vi "VisualizePmuResults.vi"() -> ()   [LabVIEW 2018, in "Visualization.lvlib" / "VisualizeAnalysis.lvclass"]
uses:
  VisualizeAnalysis.lvclass
  VisualizeBase/VisualizeBase_class/Requests/VisUserEventType.ctl
  <vilib>/event_ctls.llb/usereventprio.ctl
  <vilib>/Utility/file.llb/Read From Spreadsheet File (DBL).vi
  <vilib>/Utility/error.llb/Error Cluster From Error Code.vi
  <vilib>/ErrorRing/Error Ring.xnode
  VisualizeBase/VisualizeBase_class/VisualizeBase.lvclass
  <userlib>/NIST/NISTErrorLib/NISTErrorLib.lvlib
  Analysis/AnalysisModule/AnalysisModule.lvlib
  Visualization.lvlib
panel:
  in  "btnReset":bool
  in  "btnClear":bool
  in  "Pause":bool
  out "Data from file":dbl[][](array[numeric])
  in  "btnOpen":bool
  out "RFE":dbl(graph)=-0.0019269131938461162
  out "FE":dbl(graph)=1.1347977483922023e-05
  out "Data real time":dbl[](array[numeric])
  out "TVE":cluster{timestamp[], dbl[]}[](graph)
  in  "QueName":string="AnalVisQue"
  out "ErrorArray":errorcluster[](array[cluster])
  in  "btnStop":bool
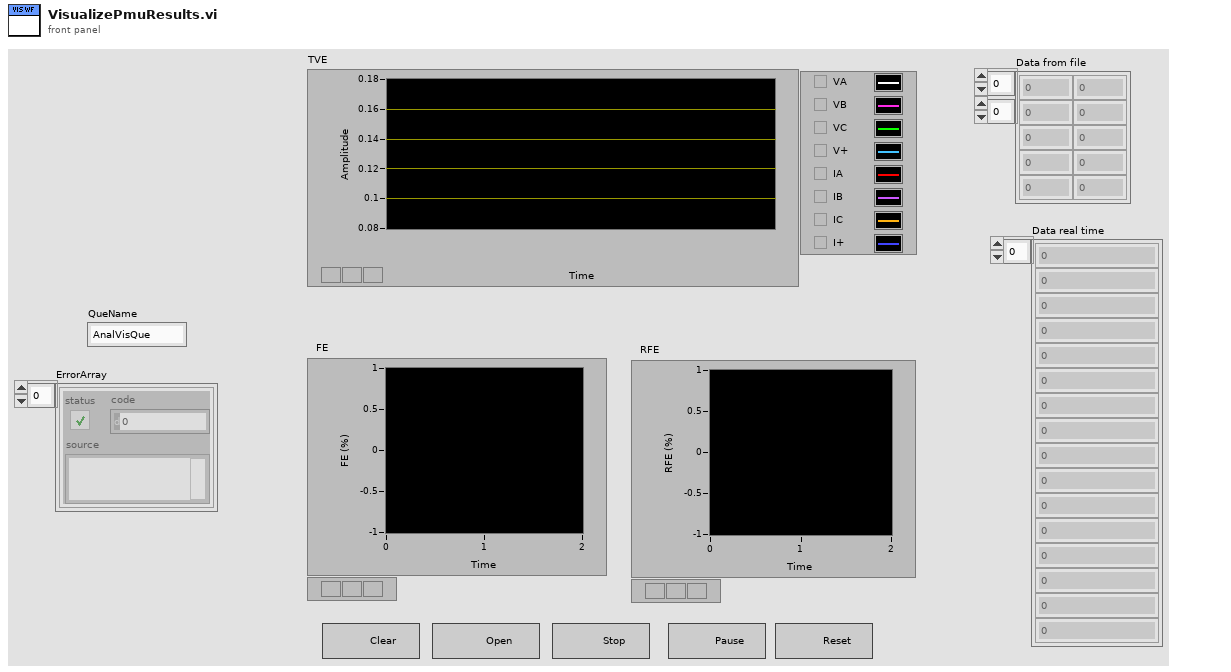
[diagram p1: front panel]
types:
  T1 = typedef "Visualization.lvlib/VisualizeBase.lvclass/VisRequestEvents.ctl" = cluster{"StopRequest":refnum<user-event>, "ResetRequest":refnum<user-event>, "FP Pop In or Out":refnum<user-event>}
  T2 = typedef "AnalysisModule.lvlib/clBroadcastEvents.ctl" = cluster{"DidInit":refnum<user-event>, "StatusUpdate":refnum<user-event>, "ErrorReport":refnum<user-event>, "DidStop":refnum<user-event>, "PathToINI":refnum<user-event>, "Config":refnum<user-event>, "ResultReport":refnum<user-event>, "FunctionClass":refnum<user-event>, "State":refnum<user-event>, "FunctionParams":refnum<user-event>, "Duration":refnum<user-event>}
  T3 = typedef "Visualization.lvlib/VisualizeBase.lvclass/VisUserEventType.ctl" = cluster{"BusIndex":i8, "Data":variant}
  T4 = typedef "usereventprio.ctl" = enum32{"high priority", "normal priority"}
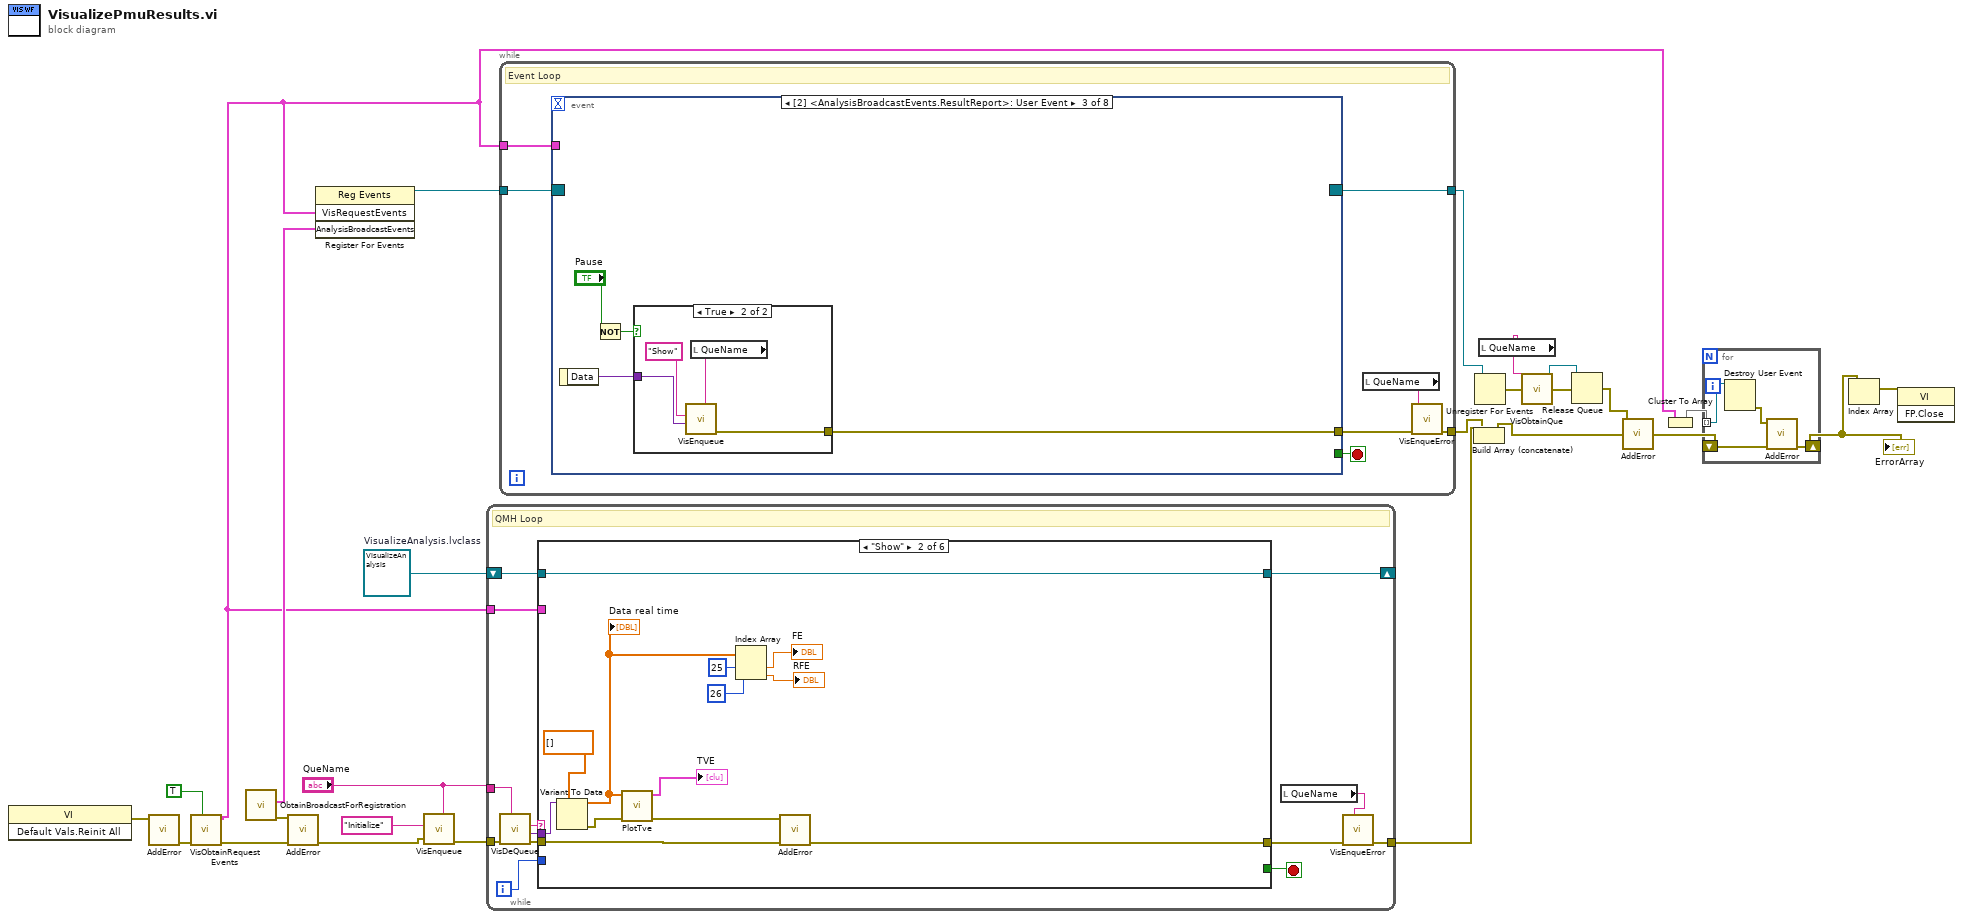
[diagram p0: block diagram]
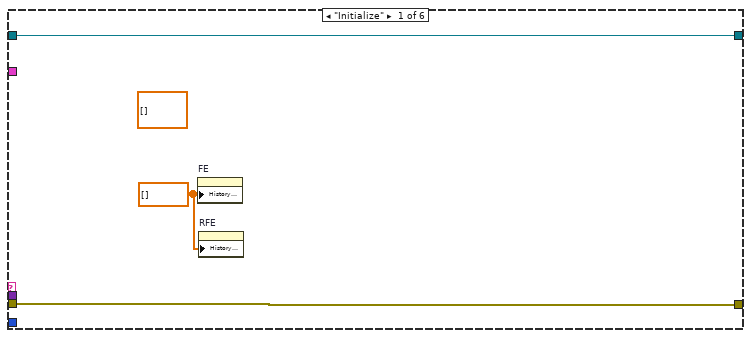
[diagram p2: hidden frame]
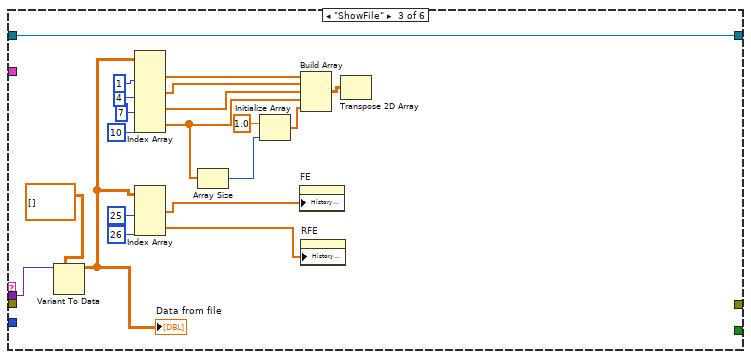
[diagram p3: hidden frame]
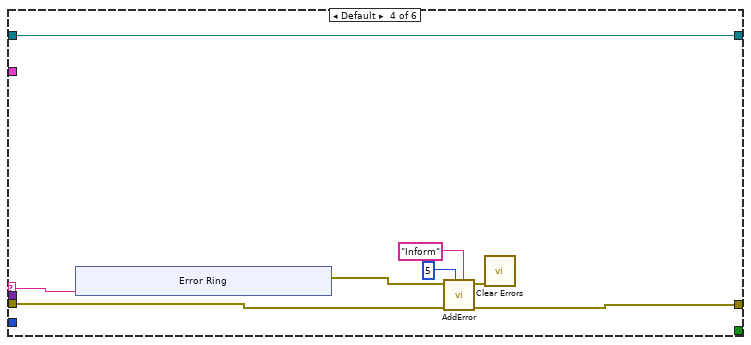
[diagram p4: hidden frame]
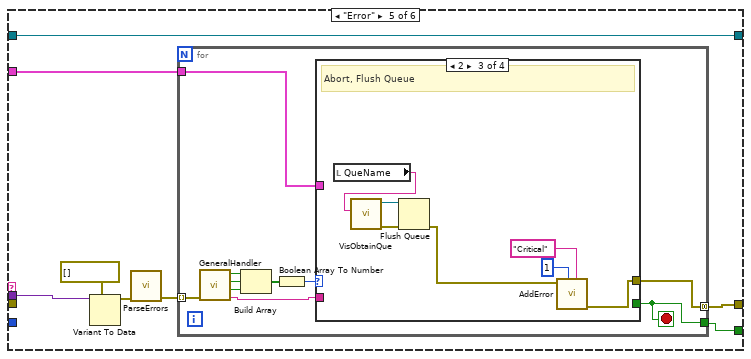
[diagram p5: hidden frame]
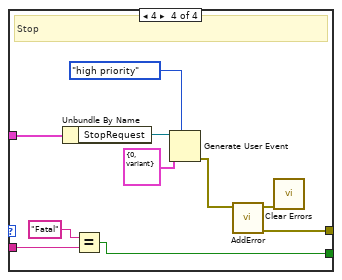
[diagram p8: hidden frame]
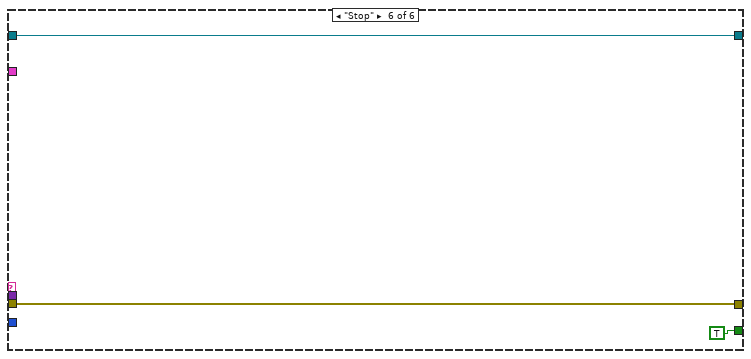
[diagram p9: hidden frame]
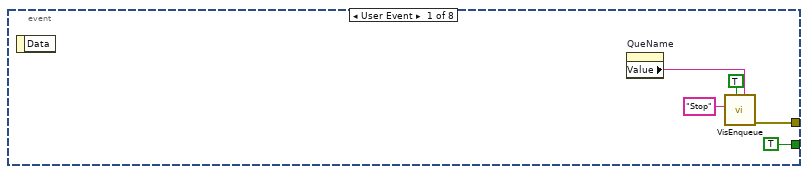
[diagram p10: hidden frame]
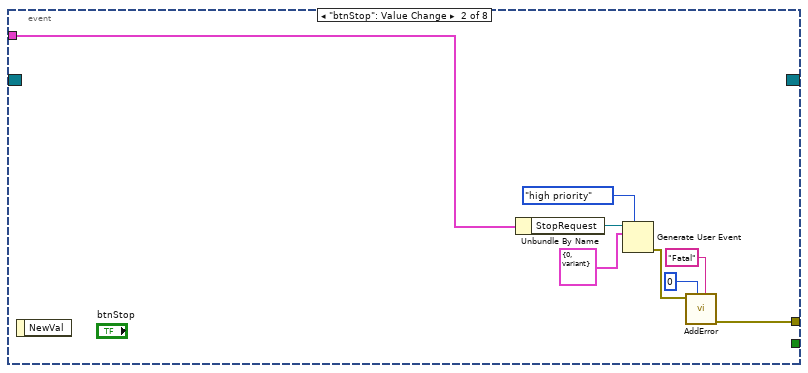
[diagram p11: hidden frame]
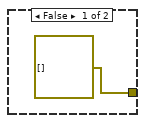
[diagram p12: hidden frame]
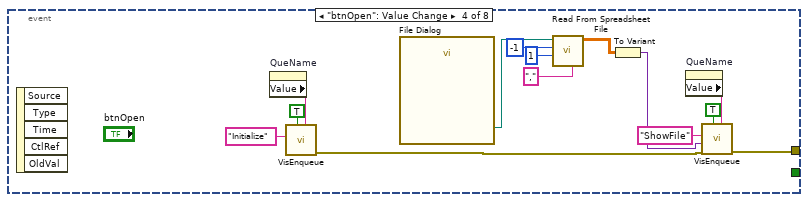
[diagram p13: hidden frame]
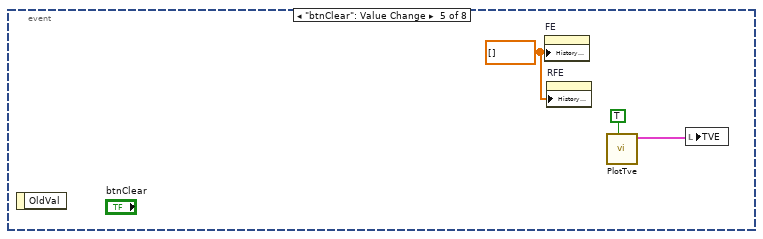
[diagram p14: hidden frame]
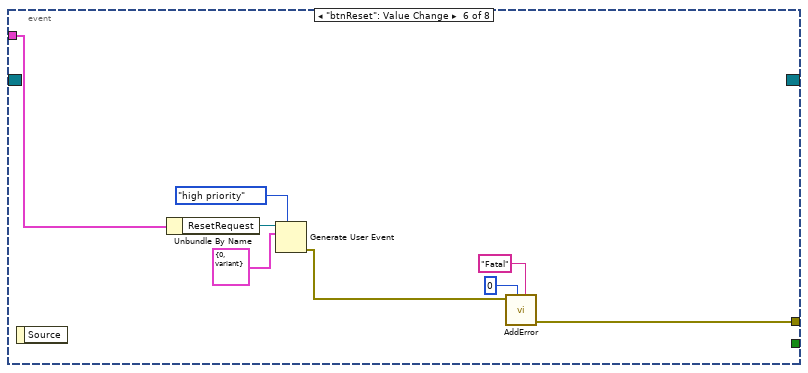
[diagram p15: hidden frame]
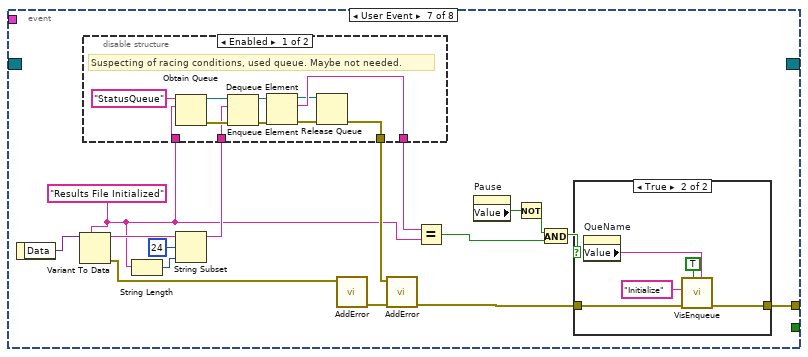
[diagram p16: hidden frame]
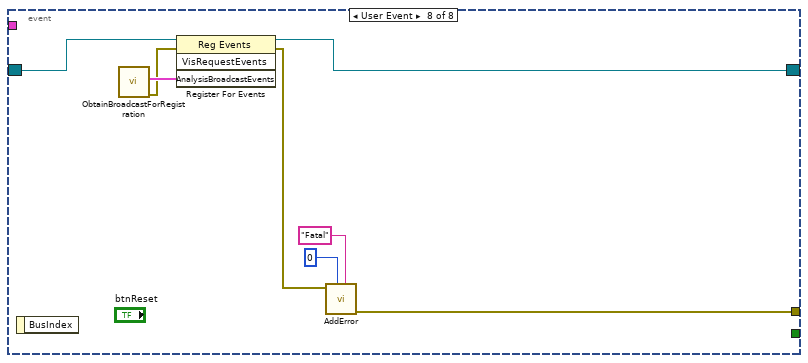
[diagram p19: hidden frame]
diagram:
  w15 = refnum<class "VisualizeAnalysis.lvclass"> refnum  # VisualizeAnalysis.lvclass
  n1 = invoke class="VI" method="Default Vals.Reinit All"() -> (error out=w22:errorcluster)  [unwired: 3 in, 2 out]
  n2 = call <userlib>:"AddError.vi"("error in (no error)"=w22) -> ("ErrorArray Out"=w21:errorcluster[])  [unwired: 9 in, 1 out]
  n3 = call "VisObtainRequestEvents.vi"("Set (T)/Get (F)"=TRUE, "Error"=w21) -> ("Error"=w19:errorcluster[], "VisRequestEvents"=w2:T1)  [unwired: 8 in]
  n4 = call "ObtainBroadcastForRegistration.vi"() -> ("error out"=w17:errorcluster, "AnalysisBroadcastEvents"=w20:T2)  [unwired: 10 in]
  n5 = call <userlib>:"AddError.vi"("ErrorArray In"=w19, "error in (no error)"=w17) -> ("ErrorArray Out"=w18:errorcluster[])  [unwired: 8 in, 1 out]
  n6 = register-events(w2, w20) -> (reference out=w14:refnum<event-registration>)  [unwired: 2 in, 1 out]
  n7 = call "VisEnqueue.vi"("QueName"="QueName", "Error"=w18, "Message"="Initialize") -> ("Error"=w25:errorcluster[])  [unwired: 8 in]
  n8 = while {
    tunnel: w25 -> [w39]
    tunnel: [w33] -> w24
    tunnel: "QueName" -> [w31]
    shift-right: [w30] -> _
    shift-left: w15 -> [w29]
    tunnel: w2 -> [w28]
    i -> [w27]
    stop <- w34 stop-if-true
    # "QMH Loop"
    n9 = call "VisDeQueue.vi"("QueName"=w31, "Error"=w39) -> ("Error"=w36:errorcluster[], "Data"=w37:variant, "Message"=w38:string)  [unwired: 7 in]
    n10 = case shown="\"Show\"" w38 {
      selector: w38 -> [_ _ _ w83 _ _]
      tunnel: w37 -> [_ w54 w75 _ w98 _]
      tunnel: w36 -> [w42 w49 _ w81 _ w127]
      tunnel: [w42 w48 _ w80 w94 w127] -> w35
      tunnel: [_ _ _ _ w93 TRUE] -> w34
      tunnel: w29 -> [w41 w55 w73 w76 w92 w126]
      tunnel: [w41 w55 w73 w76 w92 w126] -> w30
      tunnel: w28 -> [_ _ _ _ w91 _]
      tunnel: w27 -> [_ _ _ _ _ _]
      frame "Initialize" {
        w40 = dbl[] [] ("History Data")
        (unwired) dbl[][] [] ("History Data")
        n11 = property on="FE" class="WFChart (strict)"("History Data"=w40) -> ()  [unwired: 2 in, 2 out]
        n12 = property on="RFE" class="WFChart (strict)"("History Data"=w40) -> ()  [unwired: 2 in, 2 out]
      }
      frame "Show" {
        n13 = Variant To Data(type=dbl[] [], Variant=w54) -> (data=w45:dbl[], error out=w47:errorcluster)  [unwired: 1 in]
        "Data real time" <- w45
        n14 = call "PlotTve.vi"("error in (no error)"=w47, "Data real time"=w45) -> ("error out"=w46:errorcluster, "TVE"=→"TVE":cluster{timestamp[], dbl[]}[])  [unwired: 8 in]
        n15 = Index Array(array=w45, index #1=25 ("index"), index #2=26 ("index")) -> (element #1=→"FE":dbl, element #2=→"RFE":dbl)
        n16 = call <userlib>:"AddError.vi"("ErrorArray In"=w49, "error in (no error)"=w46) -> ("ErrorArray Out"=w48:errorcluster[])  [unwired: 8 in, 1 out]
      }
      frame "ShowFile" {
        n17 = Variant To Data(type=dbl[][] [], Variant=w75) -> (data=w64:dbl[][])  [unwired: 1 in, 1 out]
        "Data from file" <- w64
        n18 = Index Array(array=w64, index (col) #1=1 ("disabled index (col)"), index (col) #2=4 ("index (col)"), index (col) #3=7 ("index (col)"), index (col) #4=10 ("index (col)")) -> (element #1=w68:dbl[], element #2=w67:dbl[], element #3=w66:dbl[], element #4=w59:dbl[])  [unwired: 4 in]
        n19 = Index Array(array=w64, index (col) #1=25 ("disabled index (col)"), index (col) #2=26 ("index (col)")) -> (element #1=w61:dbl[], element #2=w60:dbl[])  [unwired: 2 in]
        n20 = Array Size(array=w59) -> (size(s)=w58:i32)
        n21 = Initialize Array(1.0 ("element"), w58) -> (w56:dbl[])
        n22 = property on="FE" class="WFChart (strict)"("History Data"=w61) -> ()  [unwired: 2 in, 2 out]
        n23 = Build Array(w68, w67, w66, w59, w56) -> (w65:dbl[][])
        n24 = property on="RFE" class="WFChart (strict)"("History Data"=w60) -> ()  [unwired: 2 in, 2 out]
        n25 = Transpose 2D Array(2D array=w65) -> ()  [unwired: 1 out]
      }
      frame Default {
        n26 = xnode "Error Ring"("parameter 0"=w83) -> ("error out"=w82:errorcluster)
        n27 = call <userlib>:"AddError.vi"("Severity"="Inform" ("String"), "Priority"=u8 5, "ErrorArray In"=w81, "error in (no error)"=w82) -> ("ErrorArray Out"=w80:errorcluster[], "error out"=w79:errorcluster)  [unwired: 6 in]
        n28 = call <vilib>:"Clear Errors.vi"("error in (no error)"=w79) -> ()  [unwired: 5 in, 2 out]
      }
      frame "Error" {
        n29 = Variant To Data(type=errorcluster[] [], Variant=w98) -> (data=w96:errorcluster[])  [unwired: 1 in, 1 out]
        n30 = call <userlib>:"ParseErrors.vi"("ErrorArray"=w96) -> ("ErrorArray"=w95:errorcluster[])  [unwired: 8 in, 2 out]
        n31 = for {
          tunnel: w95 -> [w108] mode=indexing
          tunnel: [w102] -> w94 mode=concatenating
          tunnel: [w100] -> w93
          tunnel: w91 -> [w99]
          stop <- w100 stop-if-true
          n32 = call <userlib>:"GeneralHandler.vi"("error in (no error)"=w108) -> ("Severity"=w101:string, "Stop"=w105:bool, "Abort"=w106:bool, "Continue"=w107:bool)  [unwired: 6 in, 1 out]
          n33 = Build Array(w107, w106, w105) -> (w104:bool[])
          n34 = Boolean Array To Number(Boolean array=w104) -> (number=w103:u32)
          n35 = case shown="2" w103 {
            tunnel: [_ _ w113 w124] -> w102
            tunnel: w101 -> [_ _ _ w119]
            tunnel: [_ _ _ w117] -> w100
            tunnel: w99 -> [_ _ _ w116]
            frame 0, Default {
              # "No Dialog"
            }
            frame 1 {
              # "Continue"
            }
            frame 2 {
              # "Abort, Flush Queue"
              n36 = local read "QueName"() -> (w109:string)
              n37 = call "VisObtainQue.vi"("QueName"=w109) -> ("error out"=w115:errorcluster, "queue out"=w114:refnum<queue>)  [unwired: 9 in]
              n38 = Flush Queue(queue=w114, error in (no error)=w115) -> (error out=w112:errorcluster)  [unwired: 2 out]
              n39 = call <userlib>:"AddError.vi"("Severity"="Critical" ("String"), "Priority"=u8 1, "error in (no error)"=w112) -> ("ErrorArray Out"=w113:errorcluster[])  [unwired: 7 in, 1 out]
            }
            frame 4 {
              # "Stop"
              n40 = Unbundle By Name(w116) -> ("StopRequest"=w125:refnum<user-event>)
              n41 = Equal?(x="Fatal", y=w119) -> (x = y?=w117:bool)
              n42 = Generate User Event(priority (normal)=usereventprio."high priority", user event=w125, event data cluster=T3 {"BusIndex"=0, "Data"=variant} ("event data")) -> (error out=w123:errorcluster)  [unwired: 1 in, 1 out]
              n43 = call <userlib>:"AddError.vi"("error in (no error)"=w123) -> ("ErrorArray Out"=w124:errorcluster[], "error out"=w120:errorcluster)  [unwired: 9 in]
              n44 = call <vilib>:"Clear Errors.vi"("error in (no error)"=w120) -> ()  [unwired: 5 in, 2 out]
            }
          }
        }
      }
      frame "Stop" {
      }
    }
    n45 = local read "QueName"() -> (w32:string)
    n46 = call "VisEnqueError.vi"("QueName"=w32, "Error"=w35) -> ("Error"=w33:errorcluster[])  [unwired: 9 in]
  }
  n47 = while {
    tunnel: [w133] -> w23
    tunnel: w14 -> [w131]
    tunnel: [w130] -> w8
    tunnel: w2 -> [w129]
    stop <- w135 stop-if-true
    # "Event Loop"
    n48 = event shown="[2] <AnalysisBroadcastEvents.ResultReport>: User Event" {
      selector: w131 -> [_ _ _ _ _ _ _ w217]
      dyn-events: [_ _ _ _ _ _ _ w222] -> w130
      timeout: _ -> [_ _ _ _ _ _ _ _]
      tunnel: [TRUE _ _ _ _ _ _ _] -> w135
      tunnel: [w139 w146 w151 w166 _ w175 w197 w218] -> w134
      tunnel: w129 -> [_ w141 _ _ _ w176 _ _]
      event User Event {
        n49 = event-data() -> ()  [unwired: 1 in, 1 out]
        n50 = property on="QueName" class="Str"() -> ("Value"=w136:string)  [unwired: 2 in, 2 out]
        n51 = call "VisEnqueue.vi"("QueName"=w136, "Priority? (F)"=TRUE, "Message"="Stop") -> ("Error"=w139:errorcluster[])  [unwired: 8 in]
      }
      event "btnStop": Value Change {
        n52 = event-data() -> ()  [unwired: 1 in, 1 out]
        n53 = Unbundle By Name(w141) -> ("StopRequest"=w147:refnum<user-event>)
        n54 = Generate User Event(priority (normal)=usereventprio."high priority", user event=w147, event data cluster=T3 {"BusIndex"=0, "Data"=variant} ("event data")) -> (error out=w148:errorcluster)  [unwired: 1 in, 1 out]
        n55 = call <userlib>:"AddError.vi"("Severity"="Fatal" ("String"), "Priority"=u8 0, "error in (no error)"=w148) -> ("ErrorArray Out"=w146:errorcluster[])  [unwired: 7 in, 1 out]
      }
      event User Event {
        n56 = event-data() -> ("Data"=w152:variant)  [unwired: 1 in]
        n57 = Not(x="Pause") -> (.not. x?=w149:bool)
        n58 = case shown="True" w149 {
          tunnel: w152 -> [_ w156]
          tunnel: [errorcluster[] [] ("Error") w155] -> w151
          frame False {
          }
          frame True {
            n59 = local read "QueName"() -> (w157:string)
            n60 = call "VisEnqueue.vi"("QueName"=w157, "Data"=w156, "Message"="Show") -> ("Error"=w155:errorcluster[])  [unwired: 8 in]
          }
        }
      }
      event "btnOpen": Value Change {
        n61 = event-data() -> ()  [unwired: 1 in, 5 out]
        n62 = property on="QueName" class="Str"() -> ("Value"=w163:string)  [unwired: 2 in, 2 out]
        n63 = call "VisEnqueue.vi"("QueName"=w163, "Priority? (F)"=TRUE, "Message"="Initialize") -> ("Error"=w160:errorcluster[])  [unwired: 8 in]
        n64 = call "File Dialog"() -> ("selected path"=w171:path)  [unwired: 12 in, 3 out]
        n65 = call-poly <vilib>:"Read From Spreadsheet File.vi"("delimiter (\\t)"="," ("delimiter (\\t)"), "start of read offset (chars.:0)"=1, "number of rows (all:-1)"=-1, "file path (dialog if empty)"=w171) -> ("all rows"=w165:dbl[][])  [unwired: 3 in, 4 out]
        n66 = To Variant(anything=w165) -> (Variant=w164:variant)
        n67 = property on="QueName" class="Str"() -> ("Value"=w167:string)  [unwired: 2 in, 2 out]
        n68 = call "VisEnqueue.vi"("QueName"=w167, "Priority? (F)"=TRUE, "Error"=w160, "Data"=w164, "Message"="ShowFile") -> ("Error"=w166:errorcluster[])  [unwired: 6 in]
      }
      event "btnClear": Value Change {
        w172 = dbl[] [] ("History Data")
        n69 = event-data() -> ()  [unwired: 1 in, 1 out]
        n70 = property on="FE" class="WFChart (strict)"("History Data"=w172) -> ()  [unwired: 2 in, 2 out]
        n71 = property on="RFE" class="WFChart (strict)"("History Data"=w172) -> ()  [unwired: 2 in, 2 out]
        n72 = call "PlotTve.vi"("Clear? (f)"=TRUE) -> ("TVE"=w173:cluster{timestamp[], dbl[]}[])  [unwired: 9 in, 1 out]
        n73 = local write "TVE"(w173) -> ()
      }
      event "btnReset": Value Change {
        n74 = event-data() -> ()  [unwired: 1 in, 1 out]
        n75 = Unbundle By Name(w176) -> ("ResetRequest"=w177:refnum<user-event>)
        n76 = Generate User Event(priority (normal)=usereventprio."high priority", user event=w177, event data cluster=T3 {"BusIndex"=0, "Data"=variant} ("event data")) -> (error out=w180:errorcluster)  [unwired: 1 in, 1 out]
        n77 = call <userlib>:"AddError.vi"("Severity"="Fatal", "Priority"=u8 0, "error in (no error)"=w180) -> ("ErrorArray Out"=w175:errorcluster[])  [unwired: 7 in, 1 out]
      }
      event User Event {
        w187 = "Results File Initialized" ("Status")
        n78 = event-data() -> ("Data"=w198:variant)  [unwired: 1 in]
        n79 = Variant To Data(type=w187, Variant=w198) -> (data=w195:string, error out=w192:errorcluster)  [unwired: 1 in]
        n80 = String Length(string=w187) -> (length=w188:i32)
        n81 = String Subset(string=w195, offset (0)=24, length (rest)=w188) -> (substring=w190:string)
        n82 = disable-structure shown="Enabled" {
          disable-tunnel: [w202 w210] -> w194
          disable-tunnel: [w199 _] -> w191
          disable-tunnel: w190 -> [w204 w210]
          disable-tunnel: w187 -> [w203 _]
          frame Enabled {
            # "Suspecting of racing conditions, used queue. Maybe not needed."
            n83 = Obtain Queue(name (unnamed)="StatusQueue", element data type=w203) -> (queue out=w208:refnum<queue>, error out=w206:errorcluster)  [unwired: 3 in, 1 out]
            n84 = Enqueue Element(queue=w208, element=w204, error in (no error)=w206) -> (queue out=w207:refnum<queue>, error out=w205:errorcluster)  [unwired: 1 in, 1 out]
            n85 = Dequeue Element(queue=w207, error in (no error)=w205) -> (queue out=w201:refnum<queue>, element=w202:string, error out=w200:errorcluster)  [unwired: 1 in, 1 out]
            n86 = Release Queue(queue=w201, error in (no error)=w200) -> (error out=w199:errorcluster)  [unwired: 1 in, 2 out]
          }
          frame Disabled {
          }
        }
        n87 = call <userlib>:"AddError.vi"("error in (no error)"=w192) -> ("ErrorArray Out"=w193:errorcluster[])  [unwired: 9 in, 1 out]
        n88 = call <userlib>:"AddError.vi"("ErrorArray In"=w193, "error in (no error)"=w191) -> ("ErrorArray Out"=w196:errorcluster[])  [unwired: 8 in, 1 out]
        n89 = Equal?(x=w194, y=w187) -> (x = y?=w185:bool)
        n90 = property on="Pause" class="Bool (strict)"() -> ("Value"=w184:bool)  [unwired: 2 in, 2 out]
        n91 = Not(x=w184) -> (.not. x?=w183:bool)
        n92 = And(x=w183, y=w185) -> (x .and. y?=w186:bool)
        n93 = case shown="True" w186 {
          tunnel: [w211 w213] -> w197
          tunnel: w196 -> [w211 w212]
          frame False {
          }
          frame True {
            n94 = property on="QueName" class="Str"() -> ("Value"=w214:string)  [unwired: 2 in, 2 out]
            n95 = call "VisEnqueue.vi"("QueName"=w214, "Priority? (F)"=TRUE, "Error"=w212, "Message"="Initialize") -> ("Error"=w213:errorcluster[])  [unwired: 7 in]
          }
        }
      }
      event User Event {
        n96 = event-data() -> ()  [unwired: 1 in, 1 out]
        n97 = call "ObtainBroadcastForRegistration.vi"() -> ("error out"=w223:errorcluster, "AnalysisBroadcastEvents"=w224:T2)  [unwired: 10 in]
        n98 = register-events(reference=w217, error in=w223, w224) -> (reference out=w222:refnum<event-registration>, error out=w221:errorcluster)  [unwired: 1 in]
        n99 = call <userlib>:"AddError.vi"("Severity"="Fatal", "Priority"=u8 0, "error in (no error)"=w221) -> ("ErrorArray Out"=w218:errorcluster[])  [unwired: 7 in, 1 out]
      }
    }
    n100 = local read "QueName"() -> (w132:string)
    n101 = call "VisEnqueError.vi"("QueName"=w132, "Error"=w134) -> ("Error"=w133:errorcluster[])  [unwired: 9 in]
  }
  n102 = Build Array (concatenate)(w23, w24) -> (w7:errorcluster[])
  n103 = Unregister For Events(event registration refnum=w8) -> (error out=w10:errorcluster)  [unwired: 1 in]
  n104 = local read "QueName"() -> (w4:string)
  n105 = call "VisObtainQue.vi"("error in (no error)"=w10, "QueName"=w4) -> ("error out"=w11:errorcluster, "queue out"=w12:refnum<queue>)  [unwired: 8 in]
  n106 = Release Queue(queue=w12, error in (no error)=w11) -> (error out=w13:errorcluster)  [unwired: 1 in, 2 out]
  n107 = call <userlib>:"AddError.vi"("ErrorArray In"=w7, "error in (no error)"=w13) -> ("ErrorArray Out"=w3:errorcluster[])  [unwired: 8 in, 1 out]
  n108 = Cluster To Array(cluster=w2) -> (array=w9:refnum<user-event>[])
  n109 = for {
    tunnel: w9 -> [w228] mode=indexing
    shift-right: [w227] -> w6
    shift-left: w3 -> [w226]
    n110 = Destroy User Event(user event=w228) -> (error out=w225:errorcluster)  [unwired: 1 in]
    n111 = call <userlib>:"AddError.vi"("ErrorArray In"=w226, "error in (no error)"=w225) -> ("ErrorArray Out"=w227:errorcluster[])  [unwired: 8 in, 1 out]
  }
  "ErrorArray" <- w6
  n112 = Index Array(array=w6) -> (element=w5:errorcluster)  [unwired: 1 in]
  n113 = invoke class="VI" method="FP.Close"(error in=w5) -> ()  [unwired: 2 in, 3 out]
